vi "Main Scope Sync test.vi"() -> ()   [LabVIEW 2019]
uses:
  <vilib>/rvi/eio/common/nirviEmuTemplateMethod_errors.vi
  <vilib>/eio/EIONode/EIONode.xnode
panel:
  in  "Delay":i16(ring) items=["10 ticks", "50 ticks", "1 us", "1 ms", "100 ms", "1000 ms", "1 min"]
  in  "Single DIO/Bulk DIO":bool
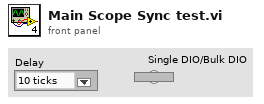
[diagram p1: front panel]
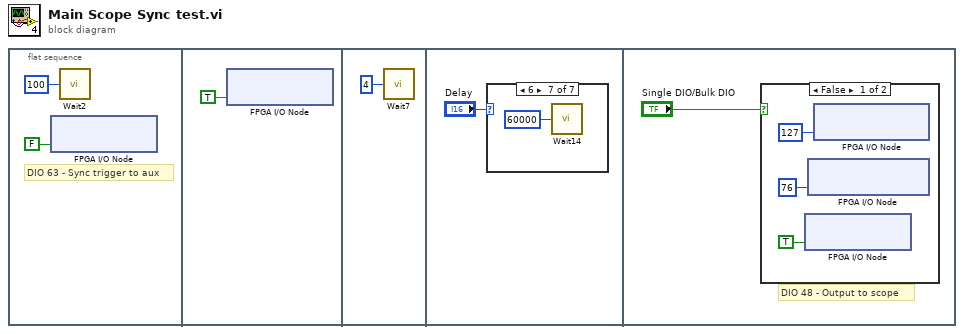
[diagram p0: block diagram]
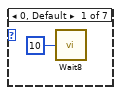
[diagram p2: hidden frame]
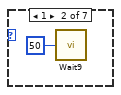
[diagram p3: hidden frame]
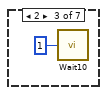
[diagram p4: hidden frame]
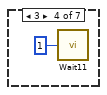
[diagram p5: hidden frame]
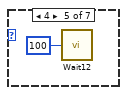
[diagram p6: hidden frame]
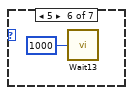
[diagram p7: hidden frame]
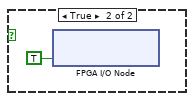
[diagram p8: hidden frame]
diagram:
  n1 = flat-sequence {
    frame #0 {
      # "DIO 63 - Sync trigger to aux"
      n2 = xnode "FPGA I/O Node"("RMC/DIO63"=FALSE) -> ()  [unwired: 1 in, 1 out]
      n3 = call "Wait2"("Count(mSec)"=u8 100) -> ()  [unwired: 1 out]
    }
    frame #1 {
      n4 = xnode "FPGA I/O Node"("RMC/DIO63"=TRUE) -> ()  [unwired: 1 in, 1 out]
    }
    frame #2 {
      n5 = call "Wait7"("Count(Ticks)"=u8 4) -> ()  [unwired: 1 out]
    }
    frame #3 {
      n6 = case shown="6" "Delay" {
        frame 0, Default {
          n7 = call "Wait8"("Count(Ticks)"=u8 10) -> ()  [unwired: 1 out]
        }
        frame 1 {
          n8 = call "Wait9"("Count(Ticks)"=u8 50) -> ()  [unwired: 1 out]
        }
        frame 2 {
          n9 = call "Wait10"("Count(uSec)"=u8 1) -> ()  [unwired: 1 out]
        }
        frame 3 {
          n10 = call "Wait11"("Count(mSec)"=u32 1) -> ()  [unwired: 1 out]
        }
        frame 4 {
          n11 = call "Wait12"("Count(mSec)"=u32 100) -> ()  [unwired: 1 out]
        }
        frame 5 {
          n12 = call "Wait13"("Count(mSec)"=u16 1000 ("Count(Ticks)")) -> ()  [unwired: 1 out]
        }
        frame 6 {
          n13 = call "Wait14"("Count(mSec)"=u16 60000 ("Count(Ticks)")) -> ()  [unwired: 1 out]
        }
      }
    }
    frame #4 {
      # "DIO 48 - Output to scope"
      n14 = case shown="False" "Single DIO/Bulk DIO" {
        frame False {
          n15 = xnode "FPGA I/O Node"("RMC/DIO48"=TRUE ("RMC/DIO47")) -> ()  [unwired: 1 in, 1 out]
          n16 = xnode "FPGA I/O Node"("RMC/DIO79:64"=u16 76) -> ()  [unwired: 1 in, 1 out]
          n17 = xnode "FPGA I/O Node"("RMC/DIO15:0"=u16 127 ("RMC/DIO79:64")) -> ()  [unwired: 1 in, 1 out]
        }
        frame True {
          n18 = xnode "FPGA I/O Node"("RMC/DIO48"=TRUE ("RMC/DIO47")) -> ()  [unwired: 1 in, 1 out]
        }
      }
    }
  }
